vi "TextDiff.vi"(8 "error in (no error)":errorcluster, 9 "Output Folders":T5, 10 "VI 2 Screenshots in":T1, 11 "VI 1 Screenshots in":T1) -> (0 "error out":errorcluster, 2 "Description":string)   [LabVIEW 2017]
uses:
  Utilities/Output Folders.ctl
  Screenshot Type.ctl
  Utilities/FilePaths.ctl
  ScreenshotInfo.ctl
  VIScreenshots.ctl
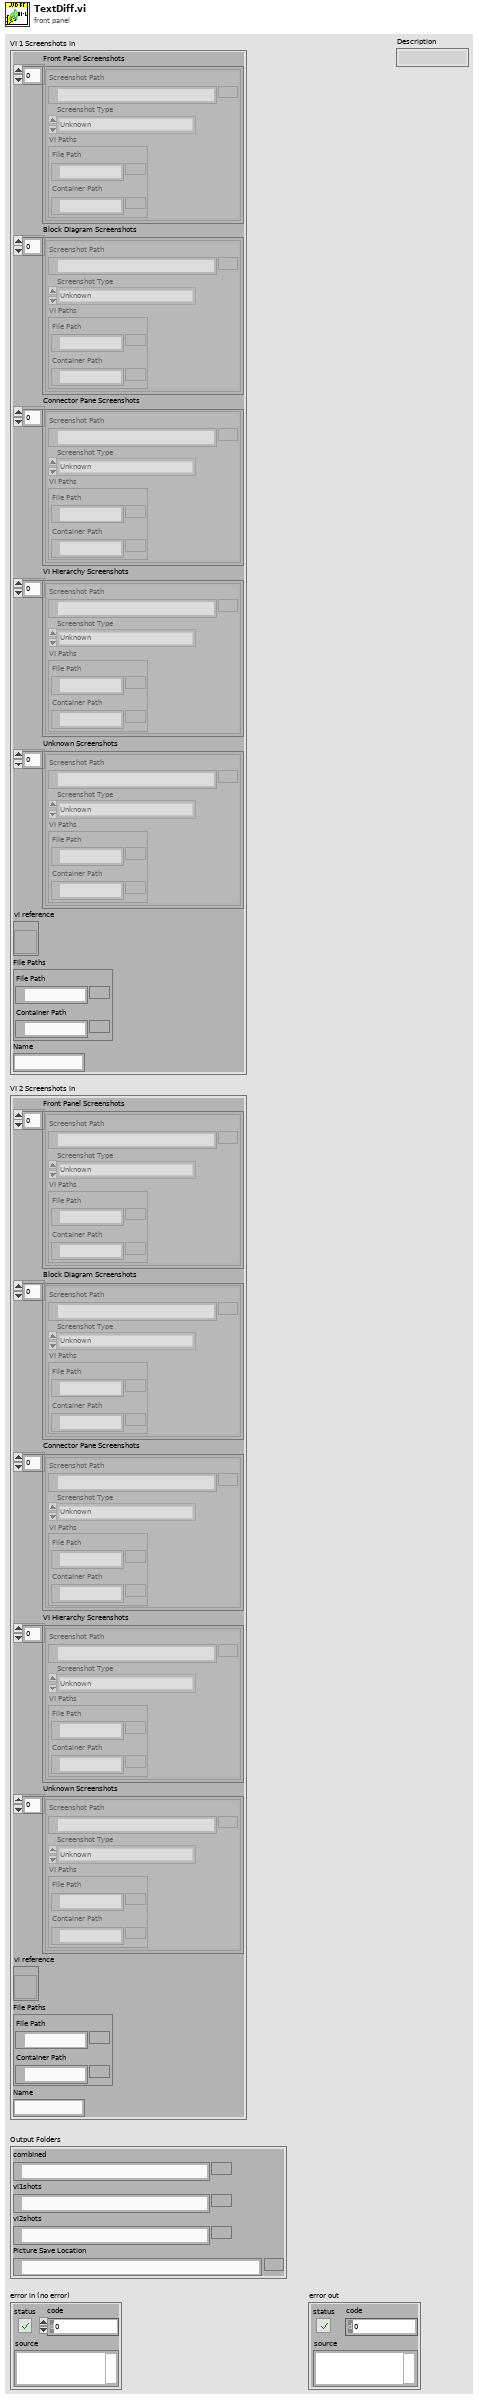
[diagram p1: front panel]
types:
  T1 = typedef "VIScreenshots.ctl" = cluster{"Front Panel Screenshots":T2[], "Block Diagram Screenshots":T2[], "Connector Pane Screenshots":T2[], "VI Hierarchy Screenshots":T2[], "Unknown Screenshots":T2[], "vi reference":refnum<vi>, "File Paths":cluster{"File Path":path, "Container Path":path}, "Name":string}
  T2 = typedef "ScreenshotInfo.ctl" = cluster{"Screenshot Path":path, "Screenshot Type":T3, "VI Paths":T4}
  T3 = typedef "Screenshot Type.ctl" = enum16{"Unknown", "Front Panel", "Connector Pane", "Block Diagram", "VI Hierarchy"}
  T4 = typedef "FilePaths.ctl" = cluster{"File Path":path, "Container Path":path}
  T5 = typedef "Output Folders.ctl" = cluster{"combined":path, "vi1shots":path, "vi2shots":path, "Picture Save Location":path}
  T6 = enum32{"invalid lock state", "Not Locked", "Locked (No Password)", "Password-protected"}
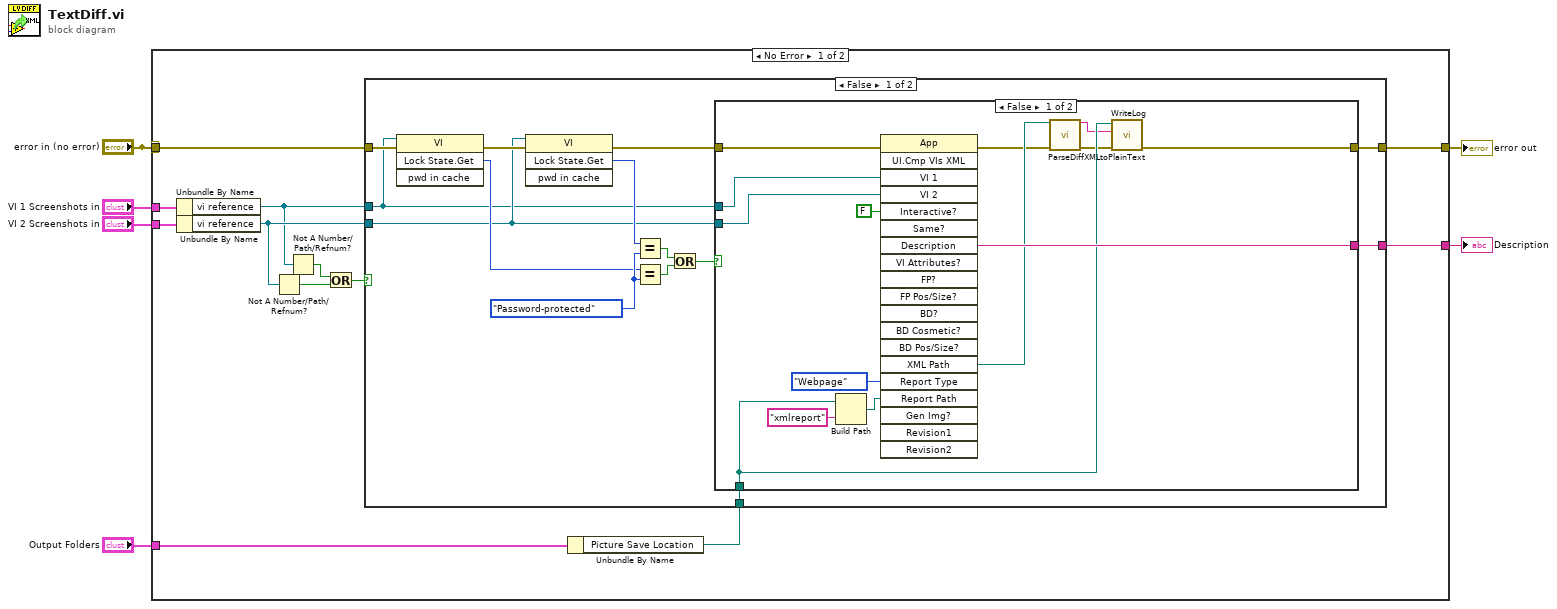
[diagram p0: block diagram]
diagram:
  n1 = case shown="No Error" "error in (no error)" {
    selector: "error in (no error)" -> [w13 w49]
    tunnel: "Output Folders" -> [w18 _]
    tunnel: "VI 2 Screenshots in" -> [w17 _]
    tunnel: "VI 1 Screenshots in" -> [w16 _]
    tunnel: "error in (no error)" -> [_ _]
    tunnel: [w15 _] -> w3
    tunnel: [w14 w49] -> w2
    frame No Error {
      n2 = Unbundle By Name(w16) -> ("vi reference"=w10:refnum<vi>)
      n3 = Unbundle By Name(w17) -> ("vi reference"=w11:refnum<vi>)
      n4 = Not A Number/Path/Refnum?(number/path/refnum=w11) -> (NaN/Path/Refnum?=w8:bool)
      n5 = Not A Number/Path/Refnum?(number/path/refnum=w10) -> (NaN/Path/Refnum?=w9:bool)
      n6 = Or(x=w9, y=w8) -> (x .or. y?=w7:bool)
      n7 = Unbundle By Name(w18) -> ("Picture Save Location"=w12:path)
      n8 = case shown="False" w7 {
        tunnel: [w32 _] -> w15
        tunnel: [w31 w48] -> w14
        tunnel: w13 -> [w30 w48]
        tunnel: w12 -> [w22 _]
        tunnel: w11 -> [w21 _]
        tunnel: w10 -> [w20 _]
        frame False {
          w27 = T6."Password-protected" ("y")
          n9 = invoke class="VI" method="Lock State.Get"(reference=w20, error in=w30) -> (error out=w28:errorcluster, "Get Lock State"=w23:T6)  [unwired: 2 in, 2 out]
          n10 = invoke class="VI" method="Lock State.Get"(reference=w21, error in=w28) -> (error out=w29:errorcluster, "Get Lock State"=w24:T6)  [unwired: 2 in, 2 out]
          n11 = Equal?(x=w24, y=w27) -> (x = y?=w25:bool)
          n12 = Equal?(x=w23, y=w27) -> (x = y?=w26:bool)
          n13 = Or(x=w25, y=w26) -> (x .or. y?=w19:bool)
          n14 = case shown="False" w19 {
            tunnel: [w46 _] -> w32
            tunnel: [w35 w47] -> w31
            tunnel: w29 -> [w45 w47]
            tunnel: w22 -> [w44 _]
            tunnel: w20 -> [w33 _]
            tunnel: w21 -> [w34 _]
            frame False {
              n15 = Build Path(base path=w44, name or relative path="xmlreport") -> (appended path=w42:path)
              n16 = invoke class="App" method="UI.Cmp VIs XML"(error in=w45, "VI 1"=w33, "VI 2"=w34, "Interactive?"=FALSE, "Report Type"=enum32{"None", "Webpage", "Text", "MS Word"}."Webpage", "Report Path"=w42) -> (error out=w36:errorcluster, "Description"=w46:string, "XML Path"=w43:path)  [unwired: 14 in, 17 out]
              n17 = call "ParseDiffXMLtoPlainText.vi"("XML Path"=w43, "error in"=w36) -> ("change description"=w38:string, "error out"=w37:errorcluster)  [unwired: 12 in]
              n18 = call "WriteLog.vi"("error in (no error)"=w37, "Log"=w38, "Log Folder"=w44) -> ("error out"=w35:errorcluster)  [unwired: 8 in]
            }
            frame True {
              # "Can't get the XML for locked VIs"
            }
          }
        }
        frame True {
        }
      }
    }
    frame Error {
    }
  }
  "Description" <- w3
  "error out" <- w2
